vi "ConditionalWhileStop.vi"() -> ()   [LabVIEW 2020]
panel:
  out "Numeric":i32
  in  "y":bool
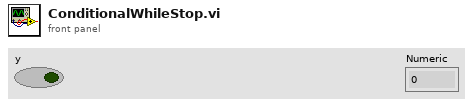
[diagram p1: front panel]
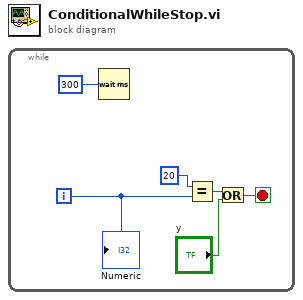
[diagram p0: block diagram]
diagram:
  n1 = while {
    i -> [w4]
    stop <- w6 stop-if-true
    n2 = Wait (ms)(milliseconds to wait=u32 300) -> ()  [unwired: 1 out]
    n3 = Equal?(x=20, y=w4) -> (x = y?=w2:bool)
    n4 = Or(x=w2, y="y") -> (x .or. y?=w6:bool)
    "Numeric" <- w4
  }
